vi "Shutdown Master.vi"(8 "error in (no error)":errorcluster, 11 "serial master in":refnum<class "Serial Master.lvclass">) -> (0 "error out":errorcluster, 3 "serial master out":refnum<class "Serial Master.lvclass">)   [LabVIEW 2018, in "SubVIs.lvlib" / "Serial Master.lvclass"]
doc: "This provides an interface for the master to close a connection to the slave."
uses:
  Serial Master.lvclass
  Serial Master.lvclass/Serial Master.ctl
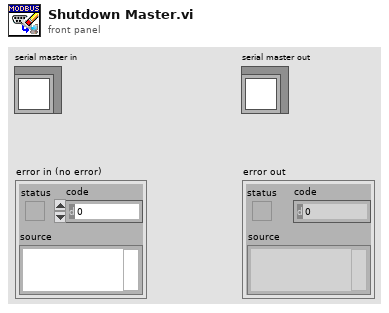
[diagram p1: front panel]
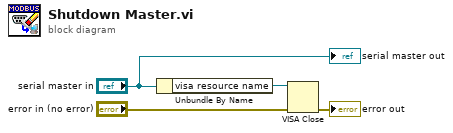
[diagram p0: block diagram]
diagram:
  n1 = Unbundle By Name("serial master in") -> ("visa resource name"=w4:refnum<visa-resource-name>)
  n2 = VISA Close(VISA resource name=w4, error in (no error)="error in (no error)") -> (error out=→"error out":errorcluster)
  "serial master out" <- "serial master in"
